vi "Configure.vi"(5 "net address":string, 7 "Multicast?":bool, 8 "error in":errorcluster, 9 "Read Timeout":i32=1000, 10 "Local Port":u16=50000) -> (0 "error out":errorcluster={"status"=TRUE, "code"=54, "source"="UDP Open in Configure.vi->EVS UDP Loop.vi"}, 3 "UDP Base out":T1={"UDP Session"=refnum, "UDP Socket Params"={"Local Port"=50000, "Read Timeout"=1000, "Write Timeout"=0}})   [LabVIEW 2011]
uses:
  UDP Base.ctl
  UDP Socket Params.ctl
  <vilib>/Utility/tcp.llb/UDP Multicast Read-Write Open.vi
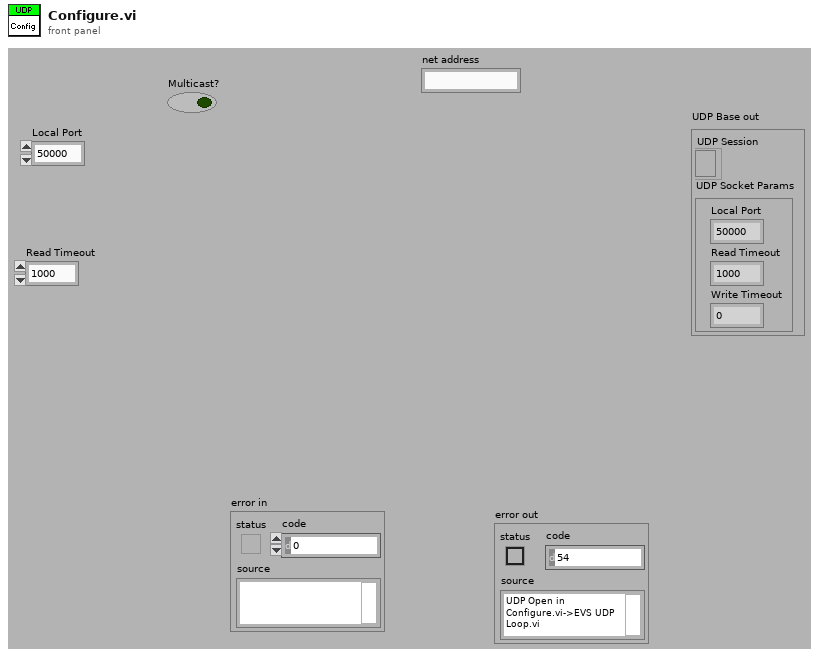
[diagram p1: front panel]
types:
  T1 = typedef "UDP Base.ctl" = cluster{"UDP Session":refnum<k16>, "UDP Socket Params":T2}
  T2 = typedef "UDP Socket Params.ctl" = cluster{"Local Port":u16, "Read Timeout":i32, "Write Timeout":i32}
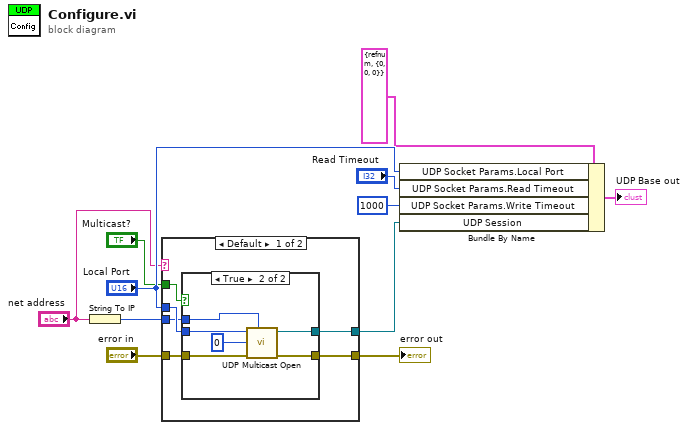
[diagram p0: block diagram]
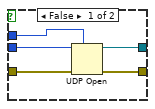
[diagram p2: hidden frame]
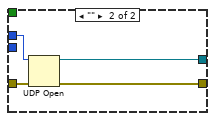
[diagram p3: hidden frame]
diagram:
  n1 = String To IP(1:"net address") -> (0:w3:u32)
  n2 = case shown="Default" "net address" {
    tunnel: "Local Port" -> [w17 w32]
    tunnel: [w16 w30] -> w10
    tunnel: "Multicast?" -> [w15 _]
    tunnel: "error in" -> [w14 w31]
    tunnel: [w13 w29] -> w6
    tunnel: w3 -> [w12 _]
    frame Default {
      n3 = case shown="True" w15 {
        tunnel: w17 -> [w21 w28]
        tunnel: [w22 w27] -> w16
        tunnel: w14 -> [w20 w26]
        tunnel: [w19 w25] -> w13
        tunnel: w12 -> [w18 w24]
        frame False {
          n4 = UDP Open(7:w18, 8:w20, 11:w21) -> (port=w19:refnum<k16>, 0:w22:errorcluster)  [unwired: 3 out]
        }
        frame True {
          n5 = call-poly <vilib>:"UDP Multicast Open.vi"("net address"=w24, "error in (no error)"=w26, "multicast addr"=u32 0, "port"=w28) -> ("error out"=w27:errorcluster, "connection ID"=w25:refnum<k16>)  [unwired: 5 in, 1 out]
        }
      }
    }
    frame "" {
      n6 = UDP Open(8:w31, 11:w32) -> (port=w29:refnum<k16>, 0:w30:errorcluster)  [unwired: 4 out]
    }
  }
  "error out" <- w10
  n7 = Bundle By Name(cluster=T1 {"UDP Session"=refnum, "UDP Socket Params"={"Local Port"=0, "Read Timeout"=0, "Write Timeout"=0}} ("UDP Base in"), "UDP Socket Params.Local Port"="Local Port", "UDP Socket Params.Read Timeout"="Read Timeout", "UDP Socket Params.Write Timeout"=1000, "UDP Session"=w6) -> (→"UDP Base out":T1)
